vi "_068.vi"   [LabVIEW 2024]
panel:
  # "Conditional Disable Structure :"
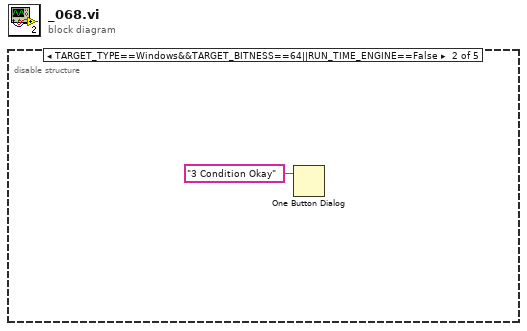
[diagram p0: block diagram]
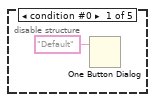
[diagram p2: hidden frame]
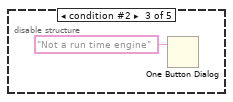
[diagram p3: hidden frame]
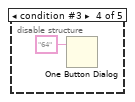
[diagram p4: hidden frame]
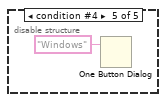
[diagram p5: hidden frame]
diagram:
  n1 = disable-structure "Conditional Disable Structure" shown="TARGET_TYPE==Windows&&TARGET_BITNESS==64||RUN_TIME_ENGINE==False" {
    frame condition #0 {
      n2 = One Button Dialog(message="Default") -> ()  [unwired: 1 in, 1 out]
    }
    frame condition #1 (active) {
      n3 = One Button Dialog(message="3 Condition Okay") -> ()  [unwired: 1 in, 1 out]
    }
    frame condition #2 {
      n4 = One Button Dialog(message="Not a run time engine") -> ()  [unwired: 1 in, 1 out]
    }
    frame condition #3 {
      n5 = One Button Dialog(message="64") -> ()  [unwired: 1 in, 1 out]
    }
    frame condition #4 {
      n6 = One Button Dialog(message="Windows") -> ()  [unwired: 1 in, 1 out]
    }
  }
